vi "SUB_run_exeFileNoWait_anyFolder.vi"(2 "exe filename":string, 3 "Base path":string) -> (0 "standard output":string, 1 "code":i32)   [LabVIEW 2011]
panel:
  out "concatenated string":string
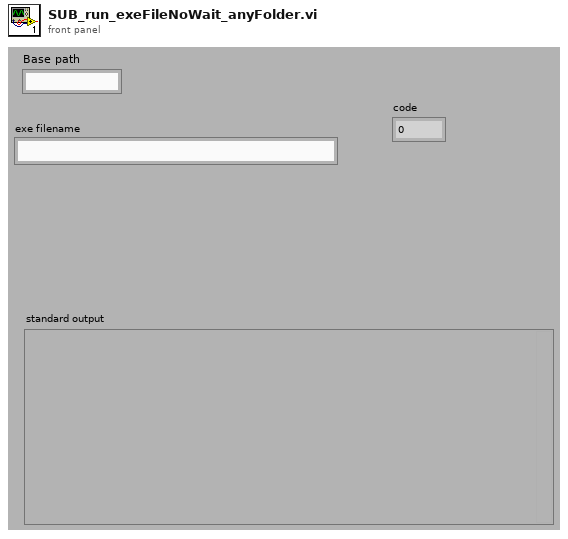
[diagram p1: front panel]
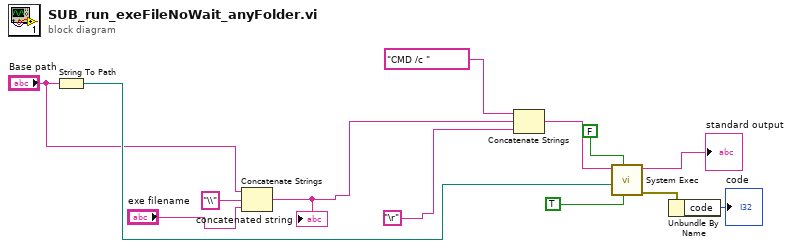
[diagram p0: block diagram]
diagram:
  n1 = String To Path(string="Base path") -> (path=w2:path)
  n2 = Concatenate Strings("Base path", "\\", "exe filename") -> (w6:string)
  "concatenated string" <- w6
  n3 = Concatenate Strings("CMD /c ", w6, "\r") -> (w11:string)
  n4 = call <vilib>:"System Exec.vi"("run minimized? (F)"=TRUE, "wait until completion? (T)"=FALSE, "working directory"=w2, "command line"=w11) -> ("error out"=w5:errorcluster, "standard output"=→"standard output":string)  [unwired: 4 in, 2 out]
  n5 = Unbundle By Name(w5) -> ("code"=→"code":i32)
